vi "Freedericksz.vi"() -> ()   [LabVIEW 2018]
uses:
  <vilib>/Utility/miscctls.llb/LVBoundsTypeDef.ctl
  <vilib>/Analysis/Matrix/Numeric/Conversions/Array To Matrix - RA.vi
  <vilib>/express/express arith-compare/Formula/XNode/ExpressFormulaBlockNode.xnode
  <vilib>/Analysis/Matrix/NI_Matrix.lvlib
panel:
  in  "Tab Control":T1(tab)
  in  "n_e":dbl=1.7 format="%#_13g"
  in  "n_o":dbl=1.5 format="%#_13g"
  out "Electric field":picture
  in  "Transition Type":u16(ring) items=["T-type"=2, "B-type"=0, "S-type"=1]
  in  "dE":dbl=0.05 min=0.0 max=2.0 step=0.01 format="%#_13g"
  in  "L - length":i32(knob)=5 min=0 max=20 step=1 scale=0.0..20.0
  in  "D - width":i32(knob)=5 min=0 step=1 scale=0.0..20.0
  in  "MCS - Monte Carlo Steps":i32=230000
  in  "dfi":dbl=0.1745 min=0.0 max=3.1415 step=0.001
  in  "check_time":i32=100
  in  "sim_time":i32=30000
  out "Fredericks transition":cluster{"Y":dbl[], "Y":dbl[]}[](graph)
  in  "stop":bool
  in  "E_endpoint":dbl=5.0 format="%#_13g"
  out "Enenrgy":cluster{"Y":dbl[], "Y":dbl[]}[](graph)
  out "LIQUID NEMATIC CRISTAL 2":picture
  in  "stop 2":bool
  in  "Order parameter \n        off/on":bool
  out "Order parameter":cluster{"Y":dbl[], "Y":dbl[]}[](graph)
  out "LIQUID NEMATIC CRISTAL":picture
  in  "Realtime simulation \n          off/on":bool
  in  "Probe_time":i32=100
  out "Current mcs step":i32
  # "The variables on the right specifies the system:\n\nL - the length in the x direction of the 2D nematic cristal, better to keep it under 20, because \n      the simulation will take too long for bigger cristals\nD - the (width) length in the y direction of the system, keep it under 20 just like the length\n\nMCS - thus are the Monte Carlo Steps, they reffer to the number  of steps (\"time steps\") the system have to \n            undergo,  let  MCS = 230000 - the default value, it is assumed that after this time the system doesn't \n             change significantly\n \nsim_time - is the number of free simulating steps, which means  the data analysis takes place after these  \n                   steps default value is 30000 (if you're in a hurry 3000 should be enuogh)\n\ncheck_time - it means we overtake the data analysis every T steps,\n                        where T is the check_time value, default: check_time=100\n\ndfi - the trying angle, which determines the new angle value in the\n         Metropolis algorythm, the best results one obtains for dfi = PI/18 = 0,1745...\n\ndE - is the electric field step (grid), the smaller the better the precision on the graph:\n\nE_endpoint - it is the endpoint of the simulation, the maximum electric field\n                     WARNING: The lower the cristal is the later the  fredericksz transition occurs, therefore the \n                                          endpoint  needs to be higher"
  # "The simulation was provided using the Metropolis algorithm for evaluating whether the change of the angle of a given molecule is\nenergetically more effective (profitable for the system). \n\nAs we can see in the above graph, the ordinary and extraordinary refraction index changes as the wavelegth of the upcoming wave rises.\nIn this simulation a constant wavlength (approximately 1800 nm - infrared) is supposed crossing an Alpha-BBO nematic liquid cristal. \nAs the electric field rises the molecules are rotating to set their orientation parallel to the field. The electric field causes the creation of \nelectric dipoles, this is why they are changing their orientation. The sudden change appears, because the dipoles interacts with each other, \nwhich causes them to keep their initialdirection. As the field gets strong enough the molecules starts to rotating and the refractive index \nchanges dus to that fact.\n \nThe sudden change in the orientation of the molecules is called the Fréedericksz transition.It is a second order \"phase\" \ntransition, which in our case is the S-type transition shown on the picture on the left. \n\nOn could at will take anothe LC cell into consideration, but it will be necessary to know the extraordinary and ordinary refractive index of that LC. As we took the Alpha-BBO cristal and used a ligth in the infrared spectrum we have these refractive indices defined as: \n(depending on the LC cell it will vary)"
  # "Now that you have a proper understanding of what this programm will show you, you can proceed \nto the next pages and watch the simulation running."
  # "Choose the transitiin type you want to observe (the types are \ndefined on the previous tab)"
  # "E_endpoint best values:\n\nD>10  -> E_end ~ 4\n4<D<10  -> E_end ~ 4,5\nD<4 -> E_end ~ 5,5"
  # "The Freedericksz transition is considered as a second order transition, because it\nfeatures a discontinuity of the second derivative in the point of the transition. \nFor such transitionsone describes the order parameter, which also features a \ndicontinuity of the second derivative at the tranition point\nThe order parameter in a nematic cristal is defined\nby the average of the Legendre polynomials as:"
  # "If you want to observe the simulation continuously or every given step (probe_time)\nthen you must consider it will take much longer to execute the whole simulation"
  # "The order parameter desribes the break of symmetry through the phase transition. In a nematic LC\nthe broken syymetry is the biaxal symmetry which shows us the graph above as the order parameter\ncrosses 0 value. As one may notice it behaves identically like the parameter which best deschribes the transition, that is the refractive index.\n\nAs we look closely on the orientation on the real time simulation of the direction of the molecules\none sees the constant oscylating in their orientation; those are thermal fluctuation. The higher the \ntemperature the heavier are those oscilations."
  # "Thanks to the simulation one could possibly derive some constants and parameters featuring the LC cell being here considered.\nOne of these characteristic constants could be the Franks splay constant and bend constant. The splay constant is directly \nrelated to the thershold electric field by the relation: (one could derive this formula minimalizing the distorion free energy):\n\n\n\n\n\nWe can see that the denominator doesn't depend on the width of the LC layer, so we can assume it at constant along the change of the width. \nComparing results for different layer widths one obtains (approximately):\n\nd = 5     ->  E_f ~ 3,3\nd = 12   ->  E_f ~ 1,25\nd = 20   ->  E_f ~ 0,75,\n\nwhere  E_f stands for the reduced (reduced parameters explained below) thershold electric field (the field as the phase transition occurs). \nLet's assume the characteristic size of the system is 'a', then we have:\n\nThis will give as an approximate value of the splay constant for the Alpha-BBO LC cell, which in terms of permittivity of vacuum and the \ncharacteristic size gives us:  \n\n\n\nSo for example for the width 15 one obtains:\n\n\nThe results are also depending on the temperature of the LC cell, but in this simulation it is assumed that the temperature is a \nquantity in the reduced parameters:\n\n\n\n\nin the hamilton function, that is:\n\n\n\n\n\n\n(The last term in this hamiltonian is not taken under consideration, because of his small influnece on the whole simulation).\nTo obtain exact values of the splay and bend constant one should add into the simulation the influence of temperature on the \nLC cell. The exact value (considering the first relation as exact) for the splay constant is then:"
  # "If one would evaulate the splay and bend conctant in a electric field under different temperatures one would obtain a curve as it is seen below, denoted with the filled black circles (the open circles reffer to simulations with a magnetic field). The upper 3 curves show the change of the bend constant and the lower ones show the splay constant. One could predict by our formula that the splay constant depends linearly on temperature, but the permittivity constant and the refractive indices depend on temperature, which wasn't earlier considered.\n\nThe results below weren't derived for the Alpha-BBO cristal, but the material that has been studied is\nthe 4-5-alkyl-4’-cyanobiphenyl compound."
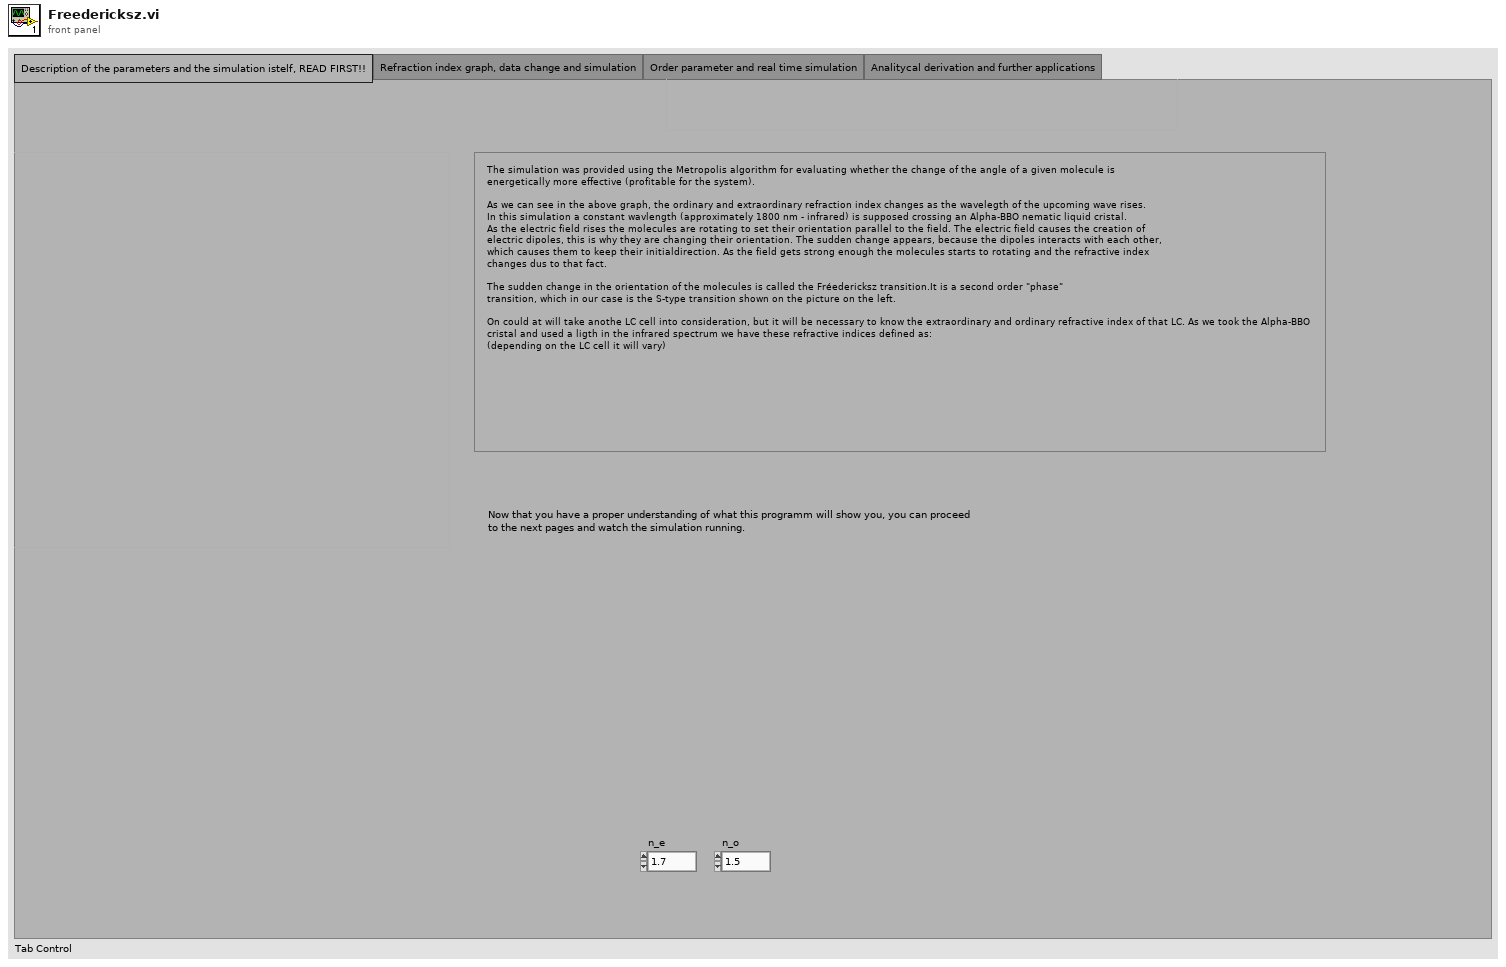
[diagram p1: front panel]
types:
  T1 = enum32{"Description of the parameters and the simulation istelf, READ FIRST!!", "Refraction index graph, data change and simulation", "Order parameter and real time simulation", "Analitycal derivation and further applications"}
  T2 = typedef "LVBoundsTypeDef.ctl" = cluster{"Width":u32, "Height":u32}
  T3 = typedef "imagedata.ctl" = cluster{"image type":i32, "image depth":i32, "image":u8[], "mask":u8[], "colors":u32[], "Rectangle":cluster{"left":i16, "top":i16, "right":i16, "bottom":i16}}
  T4 = typedef "NI_Matrix.lvlib/RealMatrix.ctl" = dbl[][]
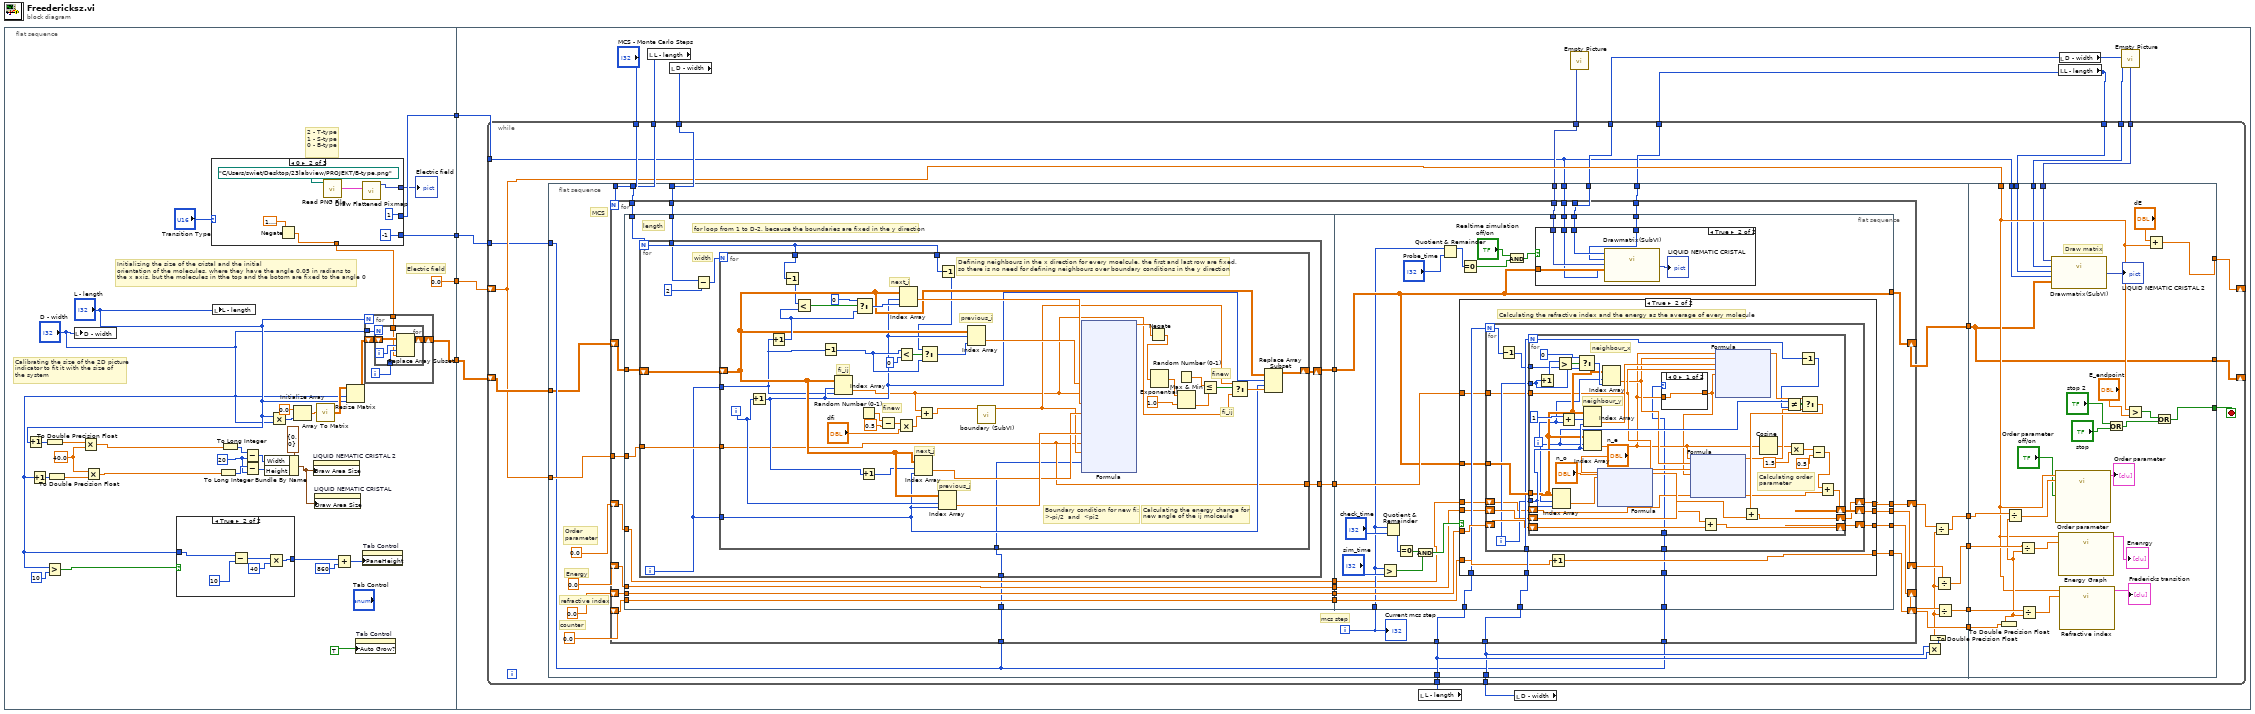
[diagram p0: block diagram]
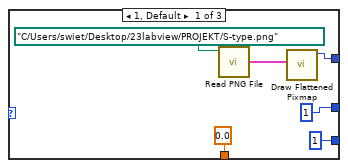
[diagram p2: hidden frame]
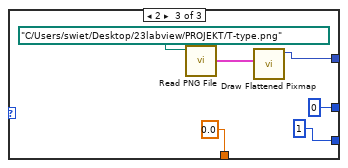
[diagram p3: hidden frame]
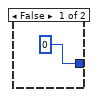
[diagram p4: hidden frame]
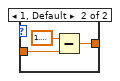
[diagram p7: hidden frame]
diagram:
  n1 = flat-sequence {
    tunnel: [0.0 ("Numeric")] -> w4
    tunnel: [w11] -> w3
    tunnel: [w13] -> w2
    tunnel: [w6] -> w1
    tunnel: w4 -> [w84]
    tunnel: w3 -> [w81]
    tunnel: w2 -> [w75]
    tunnel: w1 -> [w74]
    frame #0 {
      w22 = 20 ("y")
      w36 = 40.0 ("y")
      # "2 - T-type\n1 - S-type\n0 - B-type"
      # "Electric field"
      # "Calibrating the size of the 2D picture\nindicator to fit it with the size of\nthe system"
      # "Initializing the size of the cristal and the initial \norientation of the molecules, where they have the angle 0.05 in radians to\nthe x axis, but the molecules in tthe top and the botom are fixed to the angle 0"
      n2 = Increment(x="L - length") -> (x+1=w33:i32)
      n3 = Increment(x="D - width") -> (x+1=w32:i32)
      n4 = To Double Precision Float(number=w33) -> (double precision float=w34:dbl)
      n5 = Greater?(x="D - width", y=10) -> (0:w17:bool)
      n6 = To Double Precision Float(number=w32) -> (double precision float=w35:dbl)
      n7 = local write "D - width"("D - width") -> ()
      n8 = Multiply(x=w34, y=w36) -> (x*y=w21:dbl)
      n9 = Multiply(x=w36, y=w35) -> (x*y=w20:dbl)
      n10 = case shown="True" w17 {
        tunnel: "D - width" -> [_ w69]
        tunnel: [0 w71] -> w15
        frame False {
        }
        frame True {
          n11 = Subtract(x=w69, y=10) -> (x-y=w72:i32)
          n12 = Multiply(x=w72, y=40) -> (x*y=w71:i32)
        }
      }
      n13 = case shown="0" "Transition Type" {
        tunnel: [1 -1 1] -> w13
        tunnel: [0.0 ("element") w59 0.0] -> w7
        tunnel: [1 1 0] -> w6
        tunnel: [w49 w56 w62] -> w5
        frame 1, Default {
          n14 = call <vilib>:"Read PNG File.vi"("path to PNG file"=path "C:/Users/swiet/Desktop/23labview/PROJEKT/S-type.png") -> ("image data"=w51:T3)  [unwired: 8 in, 2 out]
          n15 = call <vilib>:"Draw Flattened Pixmap.vi"("image data"=w51) -> ("new picture"=w49:picture)  [unwired: 8 in]
        }
        frame 0 {
          n16 = Negate(x=1.5707963267948966) -> (-x=w59:dbl)
          n17 = call <vilib>:"Read PNG File.vi"("path to PNG file"=path "C:/Users/swiet/Desktop/23labview/PROJEKT/B-type.png") -> ("image data"=w57:T3)  [unwired: 8 in, 2 out]
          n18 = call <vilib>:"Draw Flattened Pixmap.vi"("image data"=w57) -> ("new picture"=w56:picture)  [unwired: 8 in]
        }
        frame 2 {
          n19 = call <vilib>:"Read PNG File.vi"("path to PNG file"=path "C:/Users/swiet/Desktop/23labview/PROJEKT/T-type.png") -> ("image data"=w64:T3)  [unwired: 8 in, 2 out]
          n20 = call <vilib>:"Draw Flattened Pixmap.vi"("image data"=w64) -> ("new picture"=w62:picture)  [unwired: 8 in]
        }
      }
      "Electric field" <- w5
      n21 = local write "L - length"("L - length") -> ()
      n22 = To Long Integer(number=w20) -> (32bit integer=w25:i32)
      n23 = To Long Integer(number=w21) -> (32bit integer=w26:i32)
      n24 = Subtract(x=w26, y=w22) -> (x-y=w23:i32)
      n25 = Subtract(x=w25, y=w22) -> (x-y=w24:i32)
      n26 = Bundle By Name(cluster=T2 {"Width"=0, "Height"=0} ("Draw Area Size"), "Width"=w23, "Height"=w24) -> (w30:T2)
      n27 = Multiply(x="L - length", y="D - width") -> (x*y=w29:i32)
      n28 = Initialize Array(0.0 ("element"), w29) -> (w28:dbl[])
      n29 = property on="LIQUID NEMATIC CRISTAL 2" class="Pict"("Draw Area Size"=w30) -> ()  [unwired: 2 in, 2 out]
      n30 = property on="LIQUID NEMATIC CRISTAL" class="Pict"("Draw Area Size"=w30) -> ()  [unwired: 2 in, 2 out]
      n31 = call-poly <vilib>:"Array To Matrix.vi"("Real 1D Array"=w28) -> ("Real Matrix (Column Vector)"=w27:T4)
      n32 = Add(x=w15, y=860) -> (x+y=w18:i32)
      n33 = Resize Matrix(1:"L - length", 2:"D - width", 4:w27) -> (0:w10:T4)
      n34 = property on="Tab Control" class="TabCtl (strict)"("Auto Grow?"=TRUE) -> ()  [unwired: 2 in, 2 out]
      n35 = property on="Tab Control" class="TabCtl (strict)"("PaneHeight"=w18) -> ()  [unwired: 2 in, 2 out]
      n36 = for {
        N: "L - length" -> [_]
        tunnel: "D - width" -> [w41]
        tunnel: w7 -> [w39]
        shift-right: [w43] -> w11
        shift-left: w10 -> [w42]
        i -> [w40]
        n37 = for {
          N: w41 -> [_]
          tunnel: w40 -> [w45]
          tunnel: w39 -> [w44]
          shift-right: [w48] -> w43
          shift-left: w42 -> [w47]
          i -> [w46]
          n38 = Replace Array Subset(array=w47, new element=w44, index (row)=w46, index (col)=w45) -> (w48:T4)
        }
      }
    }
    frame #1 {
      n39 = local read "L - length"() -> (w85:i32)
      n40 = local read "D - width"() -> (w83:i32)
      n41 = local read "L - length"() -> (w82:i32)
      n42 = local read "D - width"() -> (w86:i32)
      n43 = call "Empty Picture"() -> ("empty picture"=w79:picture)
      n44 = local read "L - length"() -> (w77:i32)
      n45 = local read "D - width"() -> (w78:i32)
      n46 = call "Empty Picture"() -> ("empty picture"=w76:picture)
      n47 = while {
        shift-right: [w95] -> _
        shift-left: w84 -> [w97]
        tunnel: w79 -> [w94]
        tunnel: "MCS - Monte Carlo Steps" -> [w107]
        tunnel: w86 -> [w104]
        tunnel: w85 -> [w106]
        tunnel: w83 -> [w100]
        tunnel: w82 -> [w105]
        tunnel: w77 -> [w103]
        tunnel: w78 -> [w102]
        shift-right: [w98] -> _
        shift-left: w81 -> [w99]
        tunnel: w78 -> [w93]
        tunnel: w77 -> [w92]
        tunnel: w76 -> [w91]
        tunnel: w75 -> [w88]
        tunnel: w74 -> [w87]
        stop <- w90 stop-if-true
        n48 = flat-sequence {
          tunnel: [w129] -> w109
          tunnel: [w131] -> w108
          tunnel: w107 -> [w135]
          tunnel: w106 -> [w124]
          tunnel: w97 -> [w132]
          tunnel: w99 -> [w111]
          tunnel: w105 -> [w127]
          tunnel: w104 -> [w126]
          tunnel: [w125] -> w101
          tunnel: w100 -> [w123]
          tunnel: [w120] -> w96
          tunnel: w94 -> [w119]
          tunnel: w93 -> [w118]
          tunnel: w92 -> [w117]
          tunnel: [w113] -> w89
          tunnel: w88 -> [w112]
          tunnel: w87 -> [w110]
          tunnel: [w413] -> w95
          tunnel: w97 -> [w405]
          tunnel: w109 -> [w419]
          tunnel: w108 -> [w418]
          tunnel: w103 -> [w400]
          tunnel: w102 -> [w401]
          tunnel: w101 -> [w398]
          tunnel: [w398] -> w98
          tunnel: w96 -> [w415]
          tunnel: w91 -> [w399]
          tunnel: [w409] -> w90
          tunnel: w89 -> [w407]
          tunnel: w87 -> [w397]
          frame #0 {
            # "Order\nparameter"
            # "Energy"
            # "refractive index"
            # "counter"
            # "MCS"
            n49 = for {
              N: w135 -> [_]
              shift-right: [w159] -> w131
              shift-left: 0.0 -> [w151]
              shift-right: [w158] -> w128
              shift-left: 0.0 -> [w155]
              tunnel: w126 -> [w163]
              tunnel: w127 -> [w162]
              tunnel: w132 -> [w161]
              shift-right: [w152] -> w125
              shift-left: w111 -> [w153]
              tunnel: w124 -> [w150]
              tunnel: w123 -> [w149]
              shift-right: [w146] -> w121
              shift-left: 0.0 -> [w147]
              tunnel: w119 -> [w144]
              tunnel: w118 -> [w143]
              tunnel: w117 -> [w142]
              shift-right: [w140] -> w116
              shift-left: 0.0 -> [w139]
              tunnel: w112 -> [w138]
              tunnel: w112 -> [w137]
              tunnel: w110 -> [w136]
              i -> [w157]
              # "mcs step"
              n50 = flat-sequence {
                tunnel: w161 -> [w174]
                tunnel: w153 -> [w173]
                tunnel: [w172] -> w160
                tunnel: w151 -> [w171]
                tunnel: [w171] -> w156
                tunnel: w155 -> [w170]
                tunnel: [w170] -> w154
                tunnel: w150 -> [w169]
                tunnel: w149 -> [w168]
                tunnel: w147 -> [w167]
                tunnel: [w167] -> w148
                tunnel: [w166] -> w145
                tunnel: w139 -> [w165]
                tunnel: [w165] -> w141
                tunnel: w138 -> [w164]
                tunnel: w163 -> [w265]
                tunnel: w162 -> [w270]
                tunnel: w160 -> [w261]
                tunnel: [w269] -> w159
                tunnel: [w268] -> w158
                tunnel: [w261] -> w152
                tunnel: w157 -> [w253]
                tunnel: w156 -> [w267]
                tunnel: w154 -> [w266]
                tunnel: w148 -> [w264]
                tunnel: [w263] -> w146
                tunnel: w145 -> [w262]
                tunnel: w144 -> [w260]
                tunnel: w143 -> [w259]
                tunnel: w142 -> [w258]
                tunnel: w141 -> [w251]
                tunnel: [w250] -> w140
                tunnel: w137 -> [w249]
                tunnel: w136 -> [w248]
                frame #0 {
                  # "for loop from 1 to D-2, because the boundaries are fixed in the y direction"
                  # "length"
                  n51 = for {
                    N: w169 -> [w184]
                    tunnel: w174 -> [w183]
                    shift-right: [w182] -> w172
                    shift-left: w173 -> [w181]
                    tunnel: w168 -> [w177]
                    tunnel: [w176] -> w166
                    tunnel: w164 -> [w175]
                    i -> [w178]
                    # "width"
                    n52 = Subtract(x=w177, y=2) -> (x-y=w180:i32)
                    n53 = for {
                      N: w180 -> [_]
                      tunnel: w178 -> [w193]
                      tunnel: w184 -> [w195]
                      tunnel: w184 -> [w194]
                      tunnel: w178 -> [w199]
                      tunnel: w183 -> [w187]
                      shift-right: [w198] -> w182
                      shift-left: w181 -> [w208]
                      tunnel: [w187] -> w176
                      tunnel: w175 -> [w185]
                      i -> [w200]
                      # "finew"
                      # "fi_ij"
                      # "Calculating the energy change for \nnew angle of the ij molceule"
                      # "Defining neighbours in the x direction for every moelcule, the first and last row are fixed, \nso there is no need for defining neighbours over boundary conditions in the y direction"
                      # "Boundary condition for new fi:\n>-pi/2  and  <pi2"
                      # "previous_j"
                      # "next_j"
                      # "fi_ij"
                      # "finew"
                      # "previous_i"
                      # "next_i"
                      n54 = Increment(x=w200) -> (x+1=w197:i32)
                      n55 = Increment(x=w193) -> (x+1=w222:i32)
                      n56 = Decrement(x=w195) -> (x-1=w196:i32)
                      n57 = Less?(x=w196, y=w222) -> (x < y?=w225:bool)
                      n58 = Decrement(x=w193) -> (x-1=w220:i32)
                      n59 = Index Array(array=w208, index (row)=w197, index (col)=w193) -> (element=w188:dbl)
                      n60 = Select(t=0, s=w225, f=w222) -> (s? t:f=w224:i32)
                      n61 = Random Number (0-1)() -> (number: 0 to 1=w219:dbl)
                      n62 = Increment(x=w197) -> (x+1=w202:i32)
                      n63 = Subtract(x=w219, y=0.5) -> (x-y=w217:dbl)
                      n64 = Multiply(x=w217, y="dfi") -> (x*y=w215:dbl)
                      n65 = Less?(x=w220, y=0) -> (x < y?=w223:bool)
                      n66 = Index Array(array=w208, index (row)=w197, index (col)=w224) -> (element=w214:dbl)
                      n67 = Index Array(array=w208, index (row)=w202, index (col)=w199) -> (element=w205:dbl)
                      n68 = Add(x=w188, y=w215) -> (x+y=w204:dbl)
                      n69 = Index Array(array=w208, index (row)=w200, index (col)=w199) -> (element=w213:dbl)
                      n70 = Decrement(x=w194) -> (x-1=w191:i32)
                      n71 = Select(t=w191, s=w223, f=w220) -> (s? t:f=w190:i32)
                      n72 = Index Array(array=w208, index (row)=w197, index (col)=w190) -> (element=w203:dbl)
                      n73 = call "boundary (SubVI).vi"("Numeric in"=w204) -> ("Numeric out"=w189:dbl)  [unwired: 10 in]
                      n74 = xnode "Formula"("fi_i"=w203, "fi_ij"=w188, "fii"=w214, "fij"=w205, "fi_j"=w213, "E"=w187, "finew"=w189, "sign"=w185) -> ("Result"=w206:dbl)  [unwired: 1 in, 1 out]
                      n75 = Negate(x=w206) -> (-x=w186:dbl)
                      n76 = Exponential ("Exponential.vi")(1:w186) -> (0:w207:dbl)
                      n77 = Random Number (0-1)() -> (number: 0 to 1=w211:dbl)
                      n78 = Max & Min(x=w207, y=1.0) -> (min(x,y)=w210:dbl)  [unwired: 1 out]
                      n79 = Less Or Equal?(x=w211, y=w210) -> (x <= y?=w209:bool)
                      n80 = Select(t=w189, s=w209, f=w188) -> (s? t:f=w201:dbl)
                      n81 = Replace Array Subset(array=w208, new element=w201, index (row)=w197, index (col)=w199) -> (w198:T4)
                    }
                  }
                }
                frame #1 {
                  n82 = Greater?(x=w253, y="sim_time") -> (0:w272:bool)
                  n83 = Quotient & Remainder(x=w253, y="check_time") -> (x-y*floor(x/y)=w274:i32)  [unwired: 1 out]
                  n84 = Equal To 0?(x=w274) -> (x = 0?=w275:bool)
                  n85 = And(x=w275, y=w272) -> (x .and. y?=w276:bool)
                  n86 = Quotient & Remainder(x=w253, y="Probe_time") -> (x-y*floor(x/y)=w257:i32)  [unwired: 1 out]
                  n87 = case shown="True" w276 {
                    tunnel: [w286 w299] -> w269
                    tunnel: w261 -> [_ w293]
                    tunnel: [w285 w295] -> w268
                    tunnel: w265 -> [_ w298]
                    tunnel: w270 -> [_ w294]
                    tunnel: w267 -> [w286 w297]
                    tunnel: w266 -> [w285 w296]
                    tunnel: w264 -> [w284 w292]
                    tunnel: [w284 w291] -> w263
                    tunnel: w262 -> [_ w290]
                    tunnel: w251 -> [w283 w289]
                    tunnel: [w283 w288] -> w250
                    tunnel: w249 -> [_ w287]
                    frame False {
                    }
                    frame True {
                      # "Calculating the refractive index and the energy as the average of every molecule"
                      n88 = for {
                        N: w294 -> [w306]
                        tunnel: w293 -> [w312]
                        shift-right: [w308] -> w295
                        shift-left: w296 -> [w310]
                        tunnel: w298 -> [w311]
                        shift-right: [w303] -> w291
                        shift-left: w292 -> [w309]
                        tunnel: w290 -> [w304]
                        shift-right: [w302] -> w288
                        shift-left: w289 -> [w301]
                        tunnel: w287 -> [w300]
                        i -> [w307]
                        n89 = Decrement(x=w306) -> (x-1=w305:i32)
                        n90 = for {
                          N: w311 -> [w343]
                          tunnel: w307 -> [w340]
                          tunnel: w312 -> [w333]
                          shift-right: [w346] -> w308
                          shift-left: w310 -> [w347]
                          shift-right: [w329] -> w303
                          shift-left: w309 -> [w328]
                          tunnel: w307 -> [w335]
                          tunnel: w305 -> [w336]
                          tunnel: w304 -> [w324]
                          shift-right: [w317] -> w302
                          shift-left: w301 -> [w316]
                          tunnel: w300 -> [w314]
                          i -> [w332]
                          # "Calculating order \nparameter"
                          # "neighbour_y"
                          # "neighbour_x"
                          n91 = Increment(x=w335) -> (x+1=w337:i32)
                          n92 = Index Array(array=w333, index (row)=w332, index (col)=w340) -> (element=w348:dbl)
                          n93 = Greater?(x=w337, y=w336) -> (0:w339:bool)
                          n94 = Add(x=1, y=w332) -> (x+y=w342:i32)
                          n95 = Select(t=0, s=w339, f=w335) -> (s? t:f=w334:i32)
                          n96 = Index Array(array=w333, index (row)=w332, index (col)=w340) -> (element=w315:dbl)
                          n97 = Index Array(array=w333, index (row)=w342, index (col)=w340) -> (element=w331:dbl)
                          n98 = xnode "Formula"("a"="n_e", "b"="n_o", "c"=w348) -> ("Result"=w327:dbl)  [unwired: 1 in, 1 out]
                          n99 = Index Array(array=w333, index (row)=w332, index (col)=w334) -> (element=w323:dbl)
                          n100 = case shown="0" w314 {
                            tunnel: w315 -> [w351 w354]
                            tunnel: [w351 w352] -> w313
                            frame 0 {
                            }
                            frame 1, Default {
                              n101 = Subtract(x=1.5707963267948966, y=w354) -> (x-y=w352:dbl)
                            }
                          }
                          n102 = xnode "Formula"("fi"=w315, "fii"=w323, "E"=w324, "alfa"=w313) -> ("Result"=w325:dbl)  [unwired: 1 in, 1 out]
                          n103 = Add(x=w327, y=w347) -> (x+y=w346:dbl)
                          n104 = xnode "Formula"("fi"=w315, "fii"=w323, "fij"=w331, "E"=w324, "alfa"=w313) -> ("Result"=w345:dbl)  [unwired: 1 in, 1 out]
                          n105 = Cosine(x=w315) -> (cos(x)=w322:dbl)
                          n106 = Multiply(x=w322, y=1.5) -> (x*y=w320:dbl)
                          n107 = Decrement(x=w343) -> (x-1=w326:i32)
                          n108 = Not Equal?(x=w332, y=w326) -> (x != y?=w344:bool)
                          n109 = Select(t=w345, s=w344, f=w325) -> (s? t:f=w330:dbl)
                          n110 = Add(x=w330, y=w328) -> (x+y=w329:dbl)
                          n111 = Subtract(x=w320, y=0.5) -> (x-y=w318:dbl)
                          n112 = Add(x=w318, y=w316) -> (x+y=w317:dbl)
                        }
                      }
                      n113 = Increment(x=w297) -> (x+1=w299:dbl)
                    }
                  }
                  n114 = Equal To 0?(x=w257) -> (x = 0?=w254:bool)
                  n115 = And(x="Realtime simulation \n          off/on", y=w254) -> (x .and. y?=w255:bool)
                  n116 = case shown="True" w255 {
                    tunnel: w261 -> [_ w278]
                    tunnel: w260 -> [_ w281]
                    tunnel: w259 -> [_ w280]
                    tunnel: w258 -> [_ w279]
                    tunnel: w248 -> [_ w277]
                    frame False {
                    }
                    frame True {
                      n117 = call "Drawmatrix(SubVI).vi"("Numeric"=w277, "Real Matrix (Column Vector)"=w278, "L - length"=w279, "D - width"=w280, "empty picture in"=w281) -> ("empty picture out"=→"LIQUID NEMATIC CRISTAL":picture)  [unwired: 6 in]
                    }
                  }
                }
              }
              "Current mcs step" <- w157
            }
            n118 = Multiply(x=w126, y=w127) -> (x*y=w130:i32)
            n119 = To Double Precision Float(number=w130) -> (double precision float=w114:dbl)
            n120 = Divide(x=w116, y=w114) -> (x/y=w113:dbl)
            n121 = Divide(x=w121, y=w114) -> (x/y=w120:dbl)
            n122 = Divide(x=w128, y=w114) -> (x/y=w129:dbl)
          }
          frame #1 {
            # "Draw matrix"
            n123 = To Double Precision Float(number=w418) -> (double precision float=w406:dbl)
            n124 = Divide(x=w407, y=w406) -> (x/y=w408:dbl)
            n125 = Divide(x=w415, y=w406) -> (x/y=w414:dbl)
            n126 = Divide(x=w419, y=w406) -> (x/y=w417:dbl)
            n127 = call "Drawmatrix(SubVI).vi"("Numeric"=w397, "Real Matrix (Column Vector)"=w398, "L - length"=w400, "D - width"=w401, "empty picture in"=w399) -> ("empty picture out"=→"LIQUID NEMATIC CRISTAL 2":picture)  [unwired: 6 in]
            n128 = call "Order parameter"("Enable"="Order parameter \n        off/on", "Y Input"=w408, "X Input"=w405) -> ("XY Graph"=→"Order parameter":cluster{"X":dbl[], "Y":dbl[]}[])  [unwired: 7 in, 1 out]
            n129 = call "Energy Graph"("Y Input"=w414, "X Input"=w405) -> ("XY Graph"=→"Enenrgy":cluster{"X":dbl[], "Y":dbl[]}[])  [unwired: 8 in, 1 out]
            n130 = call "Refractive index"("Y Input"=w417, "X Input"=w405) -> ("XY Graph"=→"Fredericks transition":cluster{"X":dbl[], "Y":dbl[]}[])  [unwired: 8 in, 1 out]
            n131 = Or(x="stop 2", y="stop") -> (x .or. y?=w412:bool)
            n132 = Greater?(x=w405, y="E_endpoint") -> (0:w421:bool)
            n133 = Add(x="dE", y=w405) -> (x+y=w413:dbl)
            n134 = Or(x=w421, y=w412) -> (x .or. y?=w409:bool)
          }
        }
      }
    }
  }
